vi "ADC SNR_Sweep_original.vi"(8 "error in (no error)":errorcluster, 9 "Sequence parameters":string[][](array[string])=[["Min limit", "Max limit", "Register sheet file", "Register Sheet"], ["", "", "CC2600.xls", "TX_BLE;Trim"], ["Reg write (addr;value)", "Operating frequency [Hz]", "", ""], ["NA", "2.44G", "", ""]], 10 "Run type":i32, 11 "Method parameters":T2={"Dev"={"Do not disturb DUT"=FALSE, "XOSC"=32000000.0, "Board type"="", "EM"="", "Configure tempboard"=TRUE, "Device specific info"=[], "Generic Object"=refnum}, "Method"={"Run type"=1, "Test name"="Current LPM2 4", "Comment"="", "Results folder"="", "AFC"=enum."Off", "Method name"="Current LPM2 4", "Method results"={"Excel brief report"=FALSE, "Spotfire report"=FALSE, "Starfish report"=FALSE}, "Operator"="", "Reference time"=timestamp(0 s since 1904-01-01), "AFC delay"=0.0, "Initialization"=enum."Enabled", "MD5 Sum"="", "HW addon board"=enum."None", "AFC Regsheet"="", "AFC Regfile"=path "", "dummy"=0.0}, "Inst"={"Instr"={"PS1"={"Name"="", "GPIB address"="", "VISA session"=""}, "PS2"={"Name"="", "GPIB address"="", "VISA session"=""}, "TC1"={"Name"="", "GPIB address"="", "VISA session"=""}, "TC2"={"Name"="", "GPIB address"="", "VISA session"=""}, "SA1"={"Name"="", "GPIB address"="", "VISA session"=""}, "SA2"={"Name"="", "GPIB address"="", "VISA session"=""}, "SG1"={"Name"="", "GPIB address"="", "VISA session"=""}, "SG2"={"Name"="", "GPIB address"="", "VISA session"=""}, "SG3"={"Name"="", "GPIB address"="", "VISA session"=""}, "MI1"={"Name"="", "GPIB address"="", "VISA session"=""}, "MI2"={"Name"="", "GPIB address"="", "VISA session"=""}, "SW SA"={"Name"="", "Controller addr"=""}, "SW SG"={"Name"="", "Controller addr"=""}, "MI3"={"Name"="", "GPIB address"="", "VISA session"=""}}, "Switchbox"={"RF Path"=0, "Cal compensation"=enum."TX", "Switchbox gain mode"="", "State"=enum."TX"}, "Instr to control (i.e. SA1)"="Default", "Intrument info string"=""}, "Sequence parameters"=[["Weight", "Min Limit", "Max Limit", "Register Sheet", "", "", "", "", "", "", "", "", ""], ["Vital", "", "1", "LPM2", "", "", "", "", "", "", "", "", ""], ["Resolution", "Reg write (addr;value)", "Chip mode", "Range", "", "", "", "", "", "", "", "", ""], ["u", "NA", "", "auto", "", "", "", "", "", "", "", "", ""]], "Cond"={"Temp logged"=25.0, "VDD1_PS1_6V"=-999.0, "VDD2_PS1_25V"=-999.0, "VDD4_PS2_25V"=-999.0, "VDD3_PS2_6V"=-999.0}, "Meas config"={"X-axis inner loop index"=32000000, "Y-axis outer loop index"=32000000, "X-axis"=[], "Y-axis"=[], "X-axis array req size"=32000000, "Y-axis array req size"=32000000, "Param description"=[], "Use meas clust for reporting"=FALSE, "Parameter index (page)"=0, "X-axis name"="", "Y-axis name"=""}} {"Cond"."VDD3_PS2_6V" format="%.3f"; "Cond"."VDD4_PS2_25V" format="%.3f"; "Cond"."VDD2_PS1_25V" format="%.3f"; "Cond"."VDD1_PS1_6V" format="%.3f"; "Method"."dummy" format="%.1p"; "Method"."AFC delay" format="%.1p"; "Dev"."XOSC" format="%.3p"}) -> (0 "Error Out":errorcluster[](array[cluster]), 1 "End Method Error":T2[](array[typedef]) {"Cond"."VDD3_PS2_6V" format="%.3f"; "Cond"."VDD4_PS2_25V" format="%.3f"; "Cond"."VDD2_PS1_25V" format="%.3f"; "Cond"."VDD1_PS1_6V" format="%.3f"; "Method"."dummy" format="%.1p"; "Method"."AFC delay" format="%.1p"; "Dev"."XOSC" format="%.3p"}, 2 "Short Results":string[](array[string]), 3 "Result summary":string[][](array[string])=[["Critical", "Output Power@2405 MHz", "-3", "4", "dBm"], ["Critical", "Output Power@2410 MHz", "-3", "4", "dBm"]])   [LabVIEW 2019]
doc: "[AutoDocStart]Performs crystal accuracy measurements. Measures the offset from ideal frequency. Primarily used for tuning XOSC capacitors and verifying XOSC trims.\n\nSweeping parameters: operating frequency, OSC override value and VDDR level\n\nResults: Offset frequency in ppm[AutoDocEnd]"
uses:
  User Lib/Generic chip methods/Classes/Generic_EM/Chameleon/Loki/Loki.lvclass
  User Lib/Generic chip methods/Classes/Generic_EM/Generic_EM/Generic_EM.lvclass
  1131283d-b54a-4ae3-ad67-71ff8f51acfe.vi
  3aacce8f-890b-4d9f-8ed2-28f84894822b.vi
  b456e919-2776-4fbb-a2ba-e4feed106c64.vi
  User Lib/Utilities/Cluster definitions/DUT VDD4.ctl
  User Lib/Utilities/Cluster definitions/DUT VDD3.ctl
  User Lib/Utilities/Cluster definitions/DUT VDD2.ctl
  User Lib/Utilities/Cluster definitions/DUT VDD1.ctl
  User Lib/Utilities/Cluster definitions/DUT vdd control.ctl
  69b5c8be-48d6-4f50-bcce-2a9f07fdba1a.vi
  User Lib/Utilities/Cluster definitions/Instr clust.ctl
  User Lib/Utilities/Cluster definitions/Method input.ctl
  User Lib/Utilities/Controls/Automatic Frequency Compensation types.ctl
  User Lib/Utilities/Controls/Method Reports.ctl
  User Lib/Utilities/Cluster definitions/Device specific info.ctl
  User Lib/Utilities/Cluster definitions/Method Initialization.ctl
  User Lib/Utilities/Switchbox control/SwitchBox_State._ENUMctl.ctl
  User Lib/Utilities/Controls/HW addon boards.ctl
panel:
  out "Output Response [All DUTs] 7":u32[][](array[numeric])
  out "Dynamic Parameters 4":T1={"SNR"=nan, "SNRD"=nan, "THD"=nan, "ENOB (SNRD)"=nan, "SFDR"=nan, "ENOB (SNR)"=nan, "Noise Power"=nan, "Signal power"=nan} {"Signal power" format="%.6f"; "Noise Power" format="%.2f"; "ENOB (SNR)" format="%.2f"; "SFDR" format="%.2f"; "ENOB (SNRD)" format="%.2f"; "THD" format="%.2f"; "SNRD" format="%.2f"; "SNR" format="%.2f"}
  out "detected Throughput":dbl=200065.4236150998
  out "Output Response [All DUTs] 6":u32[][](array[numeric])
  out "Dynamic Parameters 3":T1={"SNR"=nan, "SNRD"=nan, "THD"=nan, "ENOB (SNRD)"=nan, "SFDR"=nan, "ENOB (SNR)"=nan, "Noise Power"=nan, "Signal power"=nan} {"Signal power" format="%.6f"; "Noise Power" format="%.2f"; "ENOB (SNR)" format="%.2f"; "SFDR" format="%.2f"; "ENOB (SNRD)" format="%.2f"; "THD" format="%.2f"; "SNRD" format="%.2f"; "SNR" format="%.2f"}
  out "detected Throughput":dbl=200065.4236150998
  out "Output Response [All DUTs] 5":u32[][](array[numeric])
  out "Dynamic Parameters 2":T1={"SNR"=nan, "SNRD"=nan, "THD"=nan, "ENOB (SNRD)"=nan, "SFDR"=nan, "ENOB (SNR)"=nan, "Noise Power"=nan, "Signal power"=nan} {"Signal power" format="%.6f"; "Noise Power" format="%.2f"; "ENOB (SNR)" format="%.2f"; "SFDR" format="%.2f"; "ENOB (SNRD)" format="%.2f"; "THD" format="%.2f"; "SNRD" format="%.2f"; "SNR" format="%.2f"}
  out "detected Throughput":dbl=200065.4236150998
  out "detected Throughput":dbl=200065.4236150998
  out "Dynamic Parameters":T1={"SNR"=nan, "SNRD"=nan, "THD"=nan, "ENOB (SNRD)"=nan, "SFDR"=nan, "ENOB (SNR)"=nan, "Noise Power"=nan, "Signal power"=nan} {"Signal power" format="%.6f"; "Noise Power" format="%.2f"; "ENOB (SNR)" format="%.2f"; "SFDR" format="%.2f"; "ENOB (SNRD)" format="%.2f"; "THD" format="%.2f"; "SNRD" format="%.2f"; "SNR" format="%.2f"}
  out "Output Response [All DUTs] 4":u32[][](array[numeric])
  in  "Tab Control":T10(tab)
  # "°C"
  # "°C"
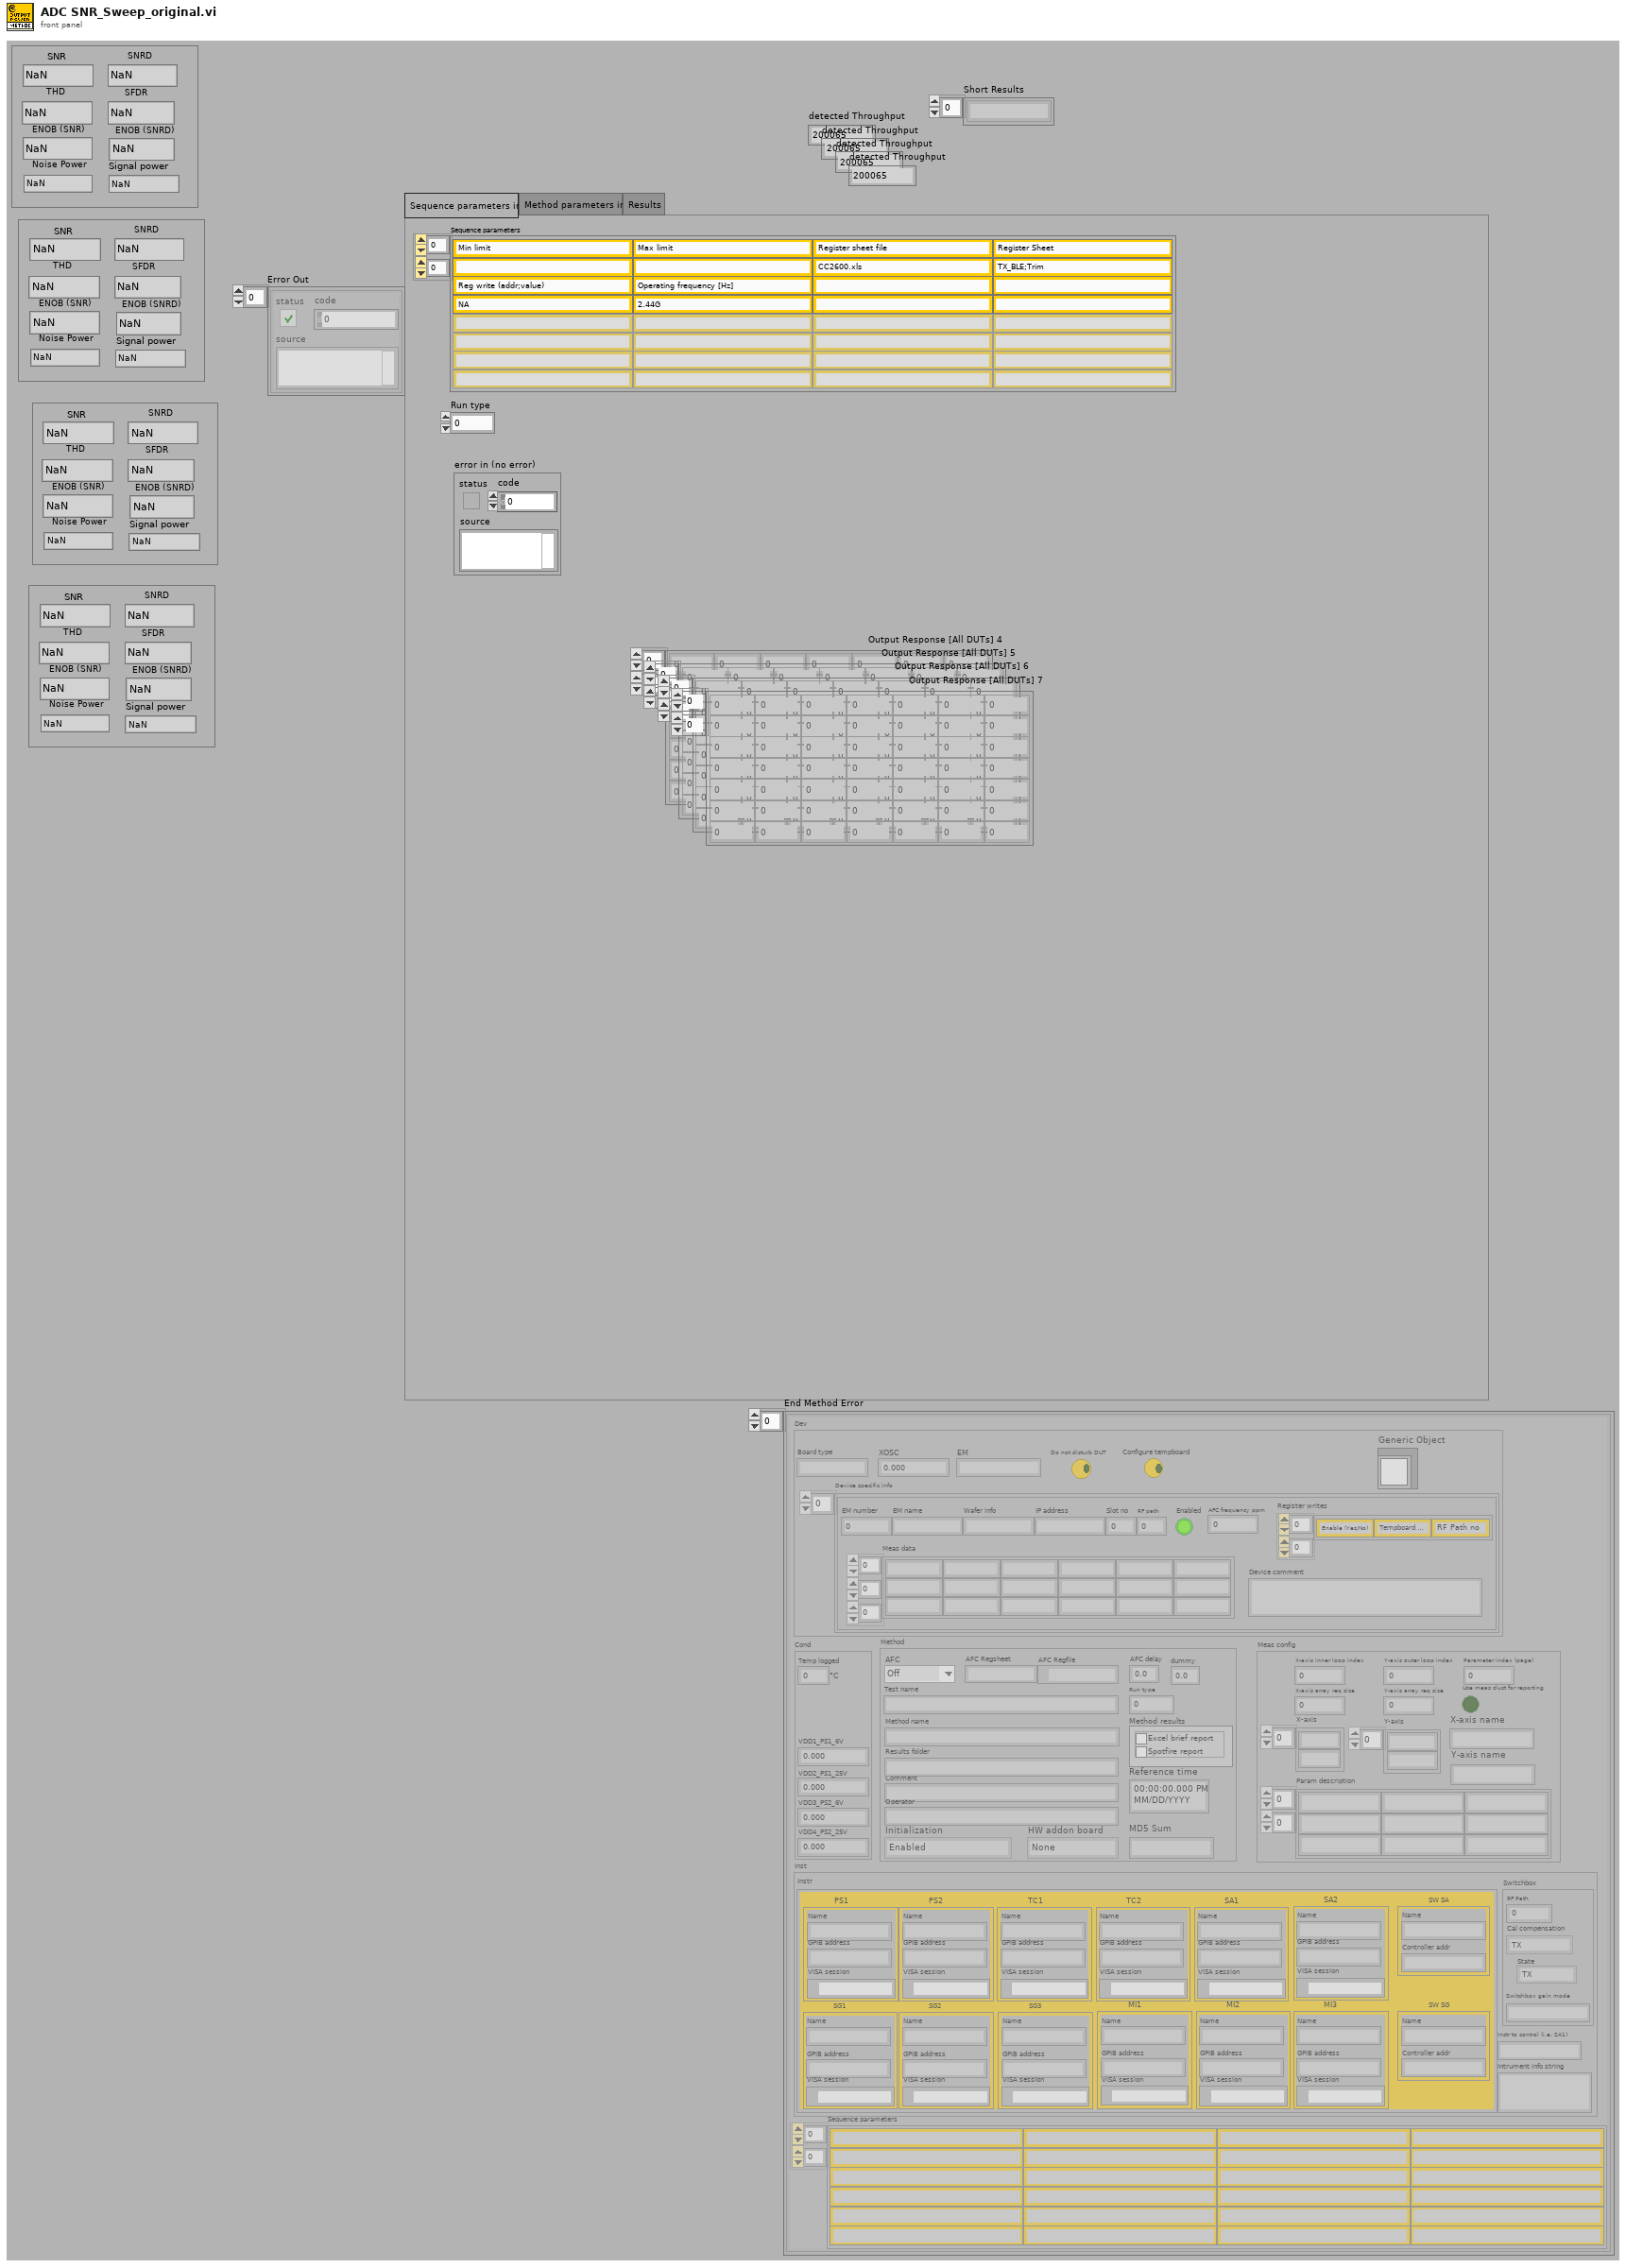
[diagram p1: front panel]
types:
  T1 = cluster{"SNR":dbl, "SNRD":dbl, "THD":dbl, "ENOB (SNRD)":dbl, "SFDR":dbl, "ENOB (SNR)":dbl, "Noise Power":dbl, "Signal power":dbl}
  T2 = typedef "Method input.ctl" = cluster{"Dev":cluster{"Do not disturb DUT":bool, "XOSC":dbl, "Board type":string, "EM":string, "Configure tempboard":bool, "Device specific info":T3[], "Generic Object":refnum<class>}, "Method":cluster{"Run type":i32, "Test name":string, "Comment":string, "Results folder":string, "AFC":T4, "Method name":string, "Method results":T5, "Operator":string, "Reference time":timestamp, "AFC delay":dbl, "Initialization":T6, "MD5 Sum":string, "HW addon board":T7, "AFC Regsheet":string, "AFC Regfile":path, "dummy":dbl}, "Inst":T8, "Sequence parameters":string[][], "Cond":cluster{"Temp logged":dbl, "VDD1_PS1_6V":dbl, "VDD2_PS1_25V":dbl, "VDD4_PS2_25V":dbl, "VDD3_PS2_6V":dbl}, "Meas config":cluster{"X-axis inner loop index":i32, "Y-axis outer loop index":i32, "X-axis":string[], "Y-axis":string[], "X-axis array req size":i32, "Y-axis array req size":i32, "Param description":string[][], "Use meas clust for reporting":bool, "Parameter index (page)":i32, "X-axis name":string, "Y-axis name":string}}
  T3 = typedef "Device specific info.ctl" = cluster{"EM number":u8, "IP address":string, "Enabled":bool, "Slot no":u8, "RF path":u8, "EM name":string, "Wafer info":string, "AFC frequency ppm":dbl, "Register writes":string[][], "Meas data":string[][][], "Device comment":string}
  T4 = typedef "Automatic Frequency Compensation types.ctl" = enum16{"Off", "Compensate Instrument frequency", "Compensate DUT frequency", "Predictive - Compensate Instrument frequency", "Predictive - Compensate DUT frequency", "Do not skip re-init - Compensate Instrument frequency", "Do not skip re-init - Compensate DUT frequency"}
  T5 = typedef "Method Reports.ctl" = cluster{"Excel brief report":bool, "Spotfire report":bool, "Starfish report":bool}
  T6 = typedef "Method Initialization.ctl" = enum16{"Enabled", "Skip Instr and Device Init", "Enabled with Separate Flash", "Set PS, Device Init and Skip Instr Init", "Skip Device Init"}
  T7 = typedef "HW addon boards.ctl" = enum16{"None", "Current meas 5EM", "Stresstest 10EM"}
  T8 = typedef "Instr clust.ctl" = cluster{"Instr":cluster{"PS1":cluster{"Name":string, "GPIB address":string, "VISA session":refnum<visa-resource-name>}, "PS2":cluster{"Name":string, "GPIB address":string, "VISA session":refnum<visa-resource-name>}, "TC1":cluster{"Name":string, "GPIB address":string, "VISA session":refnum<visa-resource-name>}, "TC2":cluster{"Name":string, "GPIB address":string, "VISA session":refnum<visa-resource-name>}, "SA1":cluster{"Name":string, "GPIB address":string, "VISA session":refnum<visa-resource-name>}, "SA2":cluster{"Name":string, "GPIB address":string, "VISA session":refnum<visa-resource-name>}, "SG1":cluster{"Name":string, "GPIB address":string, "VISA session":refnum<visa-resource-name>}, "SG2":cluster{"Name":string, "GPIB address":string, "VISA session":refnum<visa-resource-name>}, "SG3":cluster{"Name":string, "GPIB address":string, "VISA session":refnum<visa-resource-name>}, "MI1":cluster{"Name":string, "GPIB address":string, "VISA session":refnum<visa-resource-name>}, "MI2":cluster{"Name":string, "GPIB address":string, "VISA session":refnum<visa-resource-name>}, "SW SA":cluster{"Name":string, "Controller addr":string}, "SW SG":cluster{"Name":string, "Controller addr":string}, "MI3":cluster{"Name":string, "GPIB address":string, "VISA session":refnum<visa-resource-name>}}, "Switchbox":cluster{"RF Path":i32, "Cal compensation":enum16{"TX", "RX", "Interferer", "No compensation", "Interferer2"}, "Switchbox gain mode":string, "State":T9}, "Instr to control (i.e. SA1)":string, "Intrument info string":string}
  T9 = typedef "SwitchBox_State._ENUMctl.ctl" = enum16{"TX", "RX", "SP:TX", "SP:RX", "SW:TX", "SW:RX"}
  T10 = enum32{"Sequence parameters in", "Method parameters in", "Results"}
  T11 = typedef "DUT vdd control.ctl" = cluster{"VDD4 config":T12, "VDD3 config":T13, "VDD2 config":T14, "VDD1 config":T15}
  T12 = typedef "DUT VDD4.ctl" = u16
  T13 = typedef "DUT VDD3.ctl" = u16
  T14 = typedef "DUT VDD2.ctl" = u16
  T15 = typedef "DUT VDD1.ctl" = u16
  T16 = cluster{"Fundamental Frequency":dbl, "Sampling Frequncy":dbl, "No of Harmonics":u8, "Window":enum16{"None ", "Hanning", "Hamming", "Blackman-Harris", "Exact Blackman", "Blackman", "Flat Top", "4 Term B-Harris ", "7 Term B-Harris"}, "Blackman (fundamental power) bins)":dbl}
  T17 = enum32{"NI Card Settings", "Memory Read Setting", "DC Capture", "ADC Ramp", "ADC Sine", "SNR", "Cap Calibration"}
  T18 = enum32{"Read from Memory", "Read .dat file", "NI Card Capture", "None"}
  T19 = typedef "TFW ResponseData.ctl" = cluster{"errorCode":u32, "executionTime":u32, "processedCmdWord":u32, "responsePar":u32[], "actionCode":u32, "cmdStatus":u16}
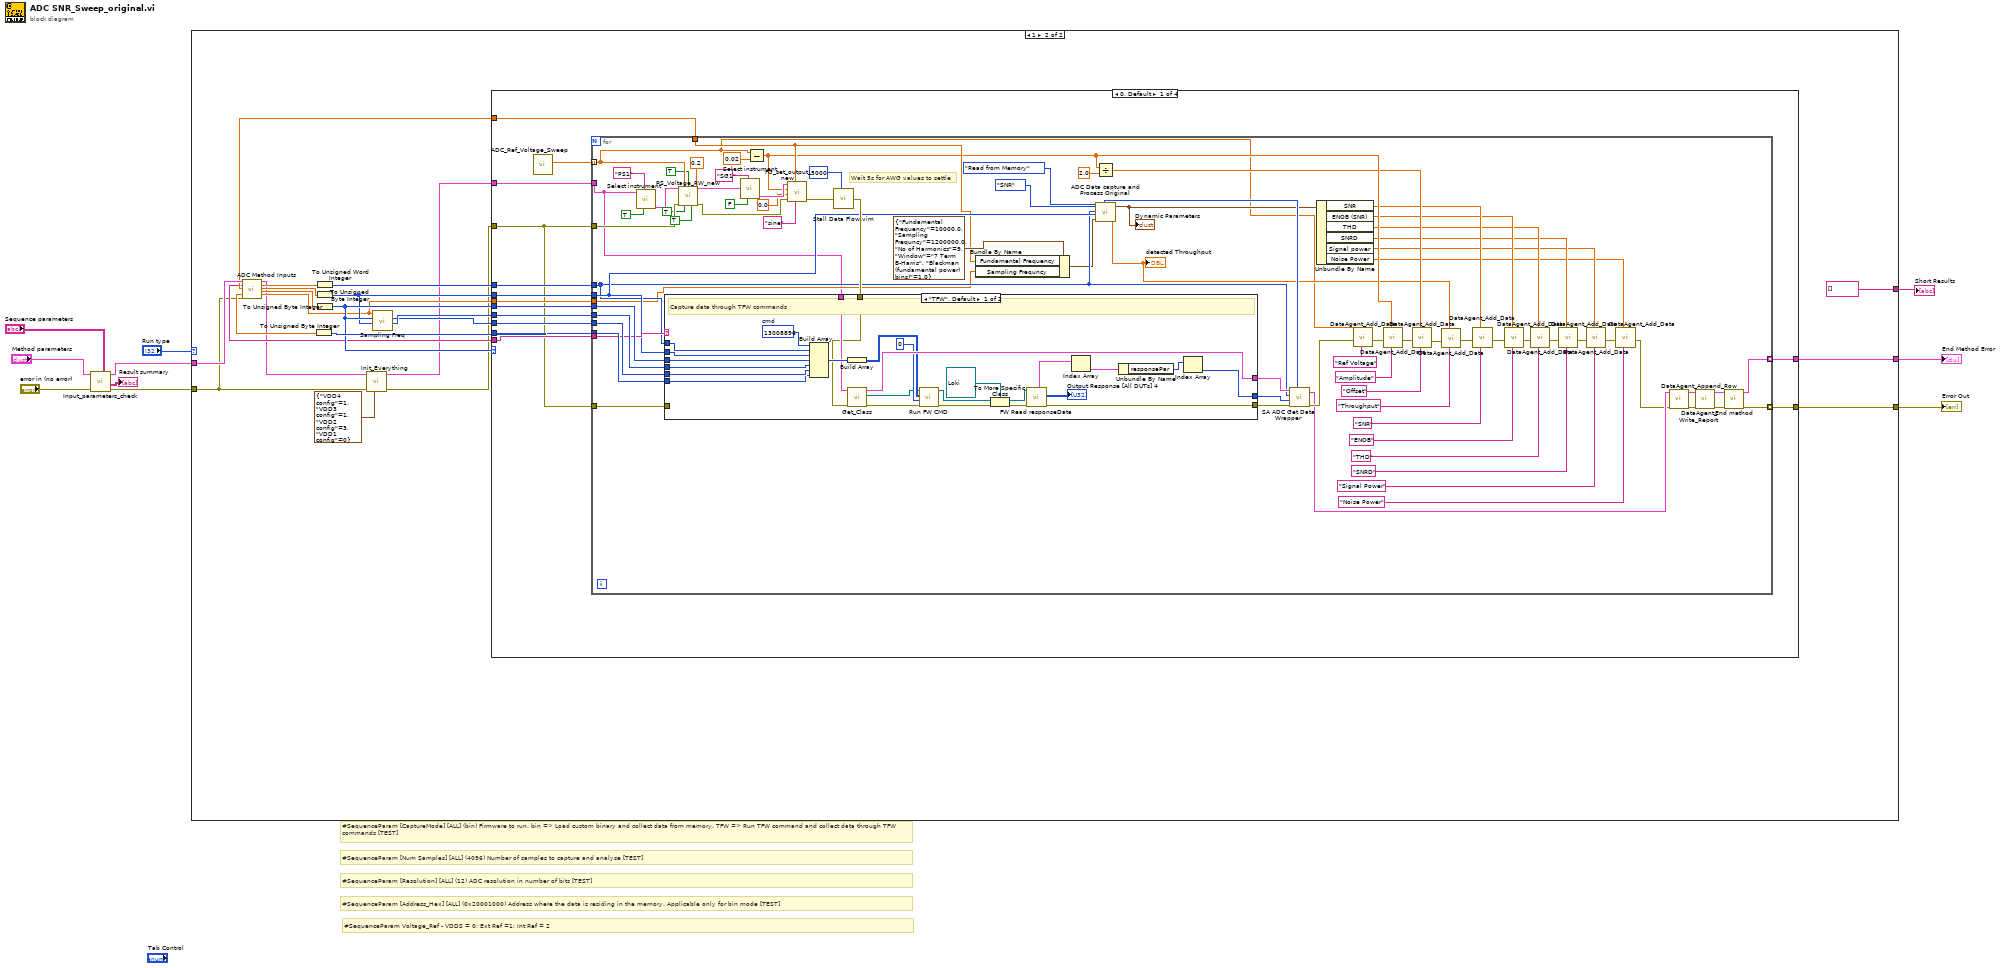
[diagram p0: block diagram]
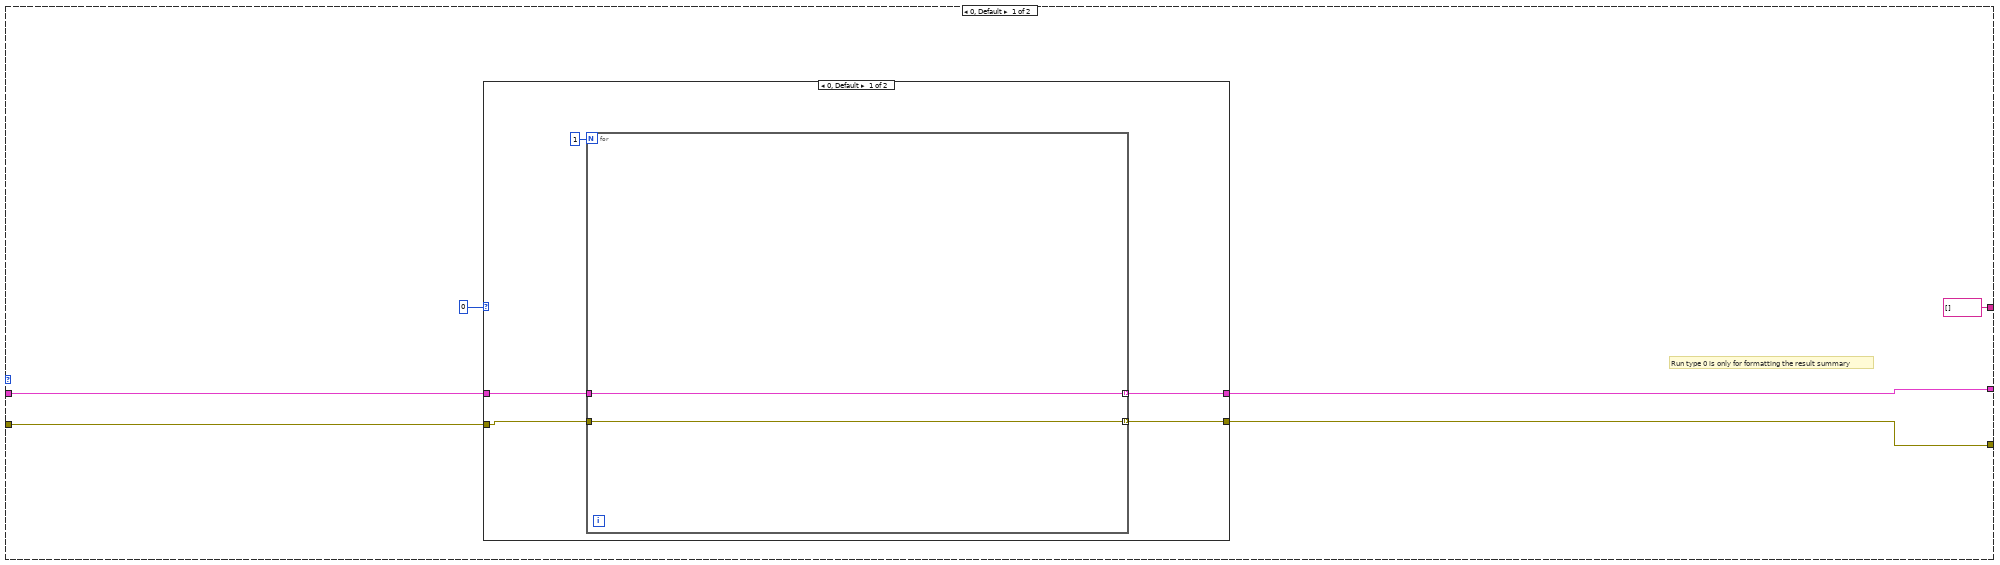
[diagram p2: hidden frame]
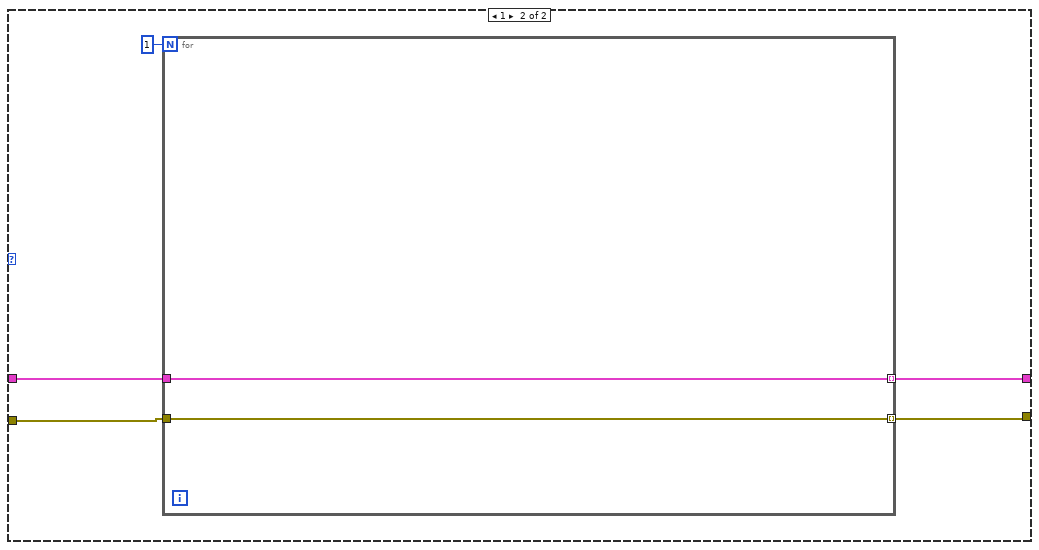
[diagram p3: hidden frame]
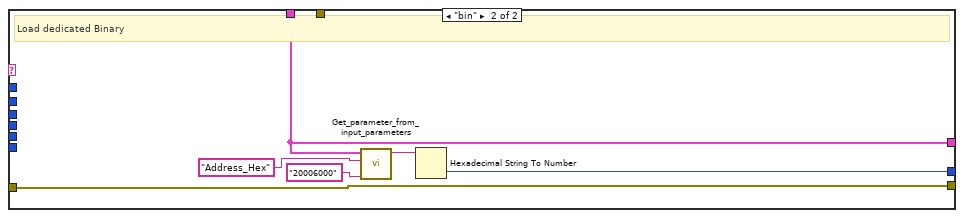
[diagram p4: hidden frame]
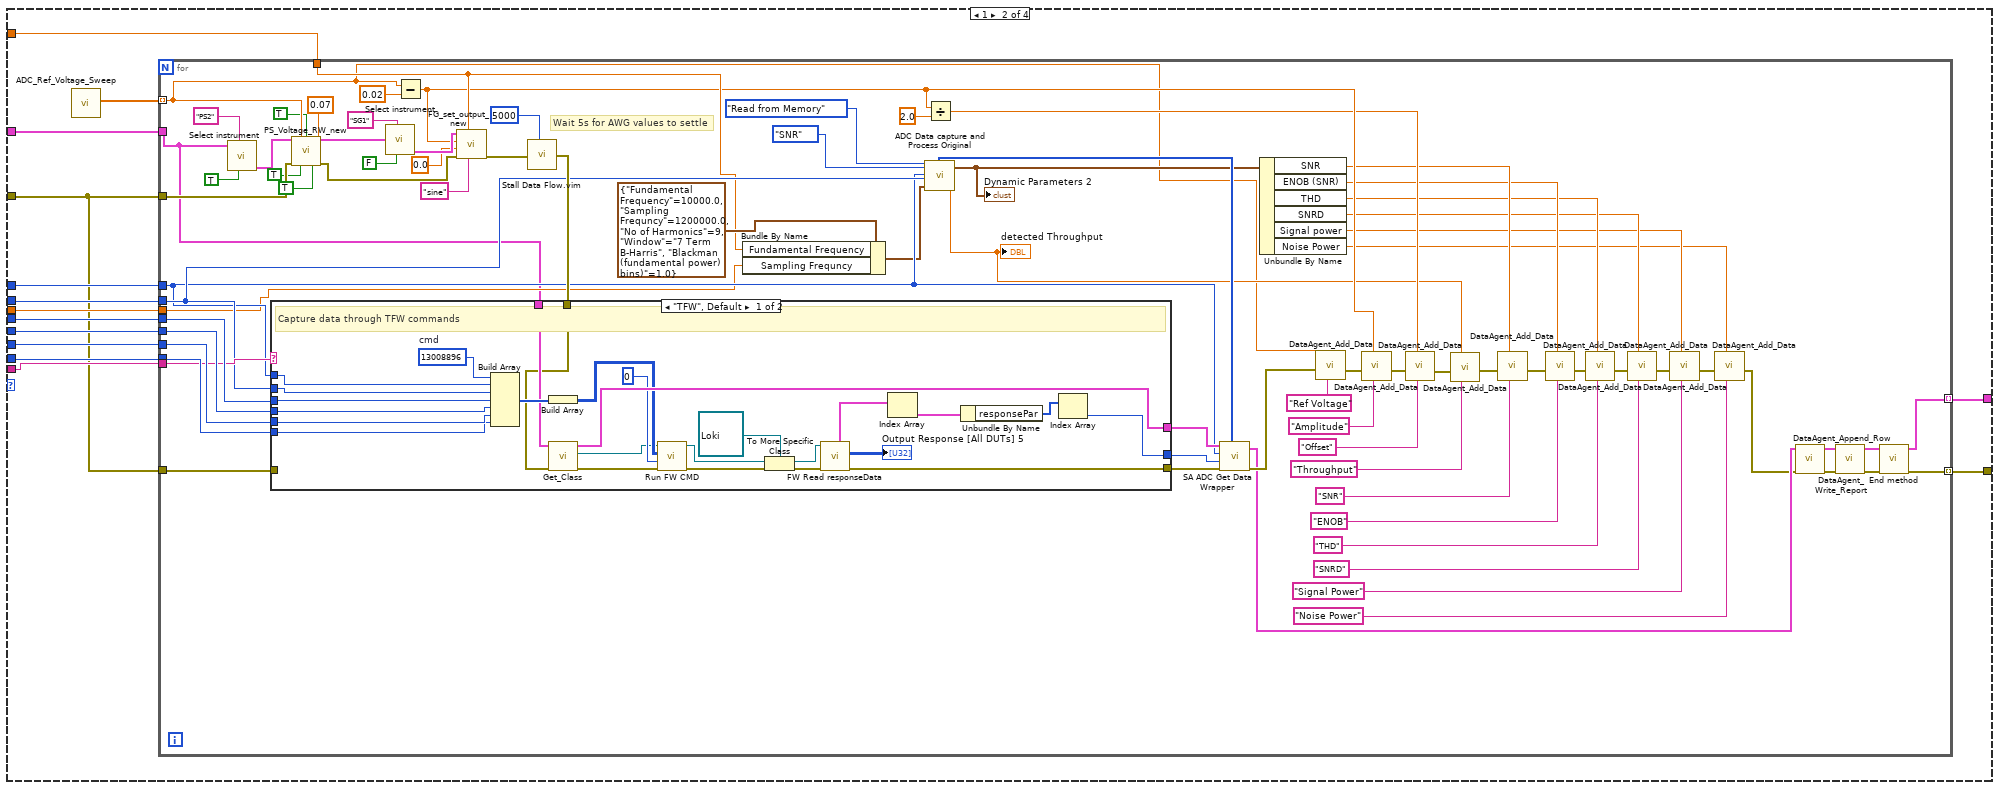
[diagram p5: hidden frame]
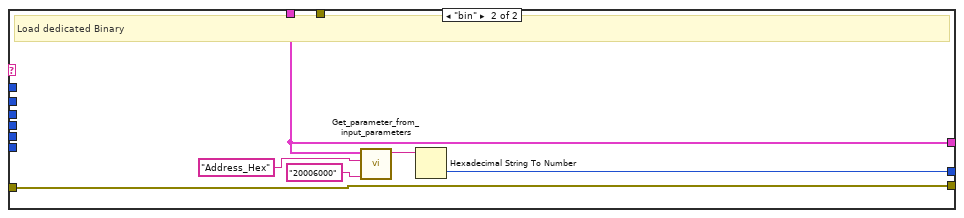
[diagram p6: hidden frame]
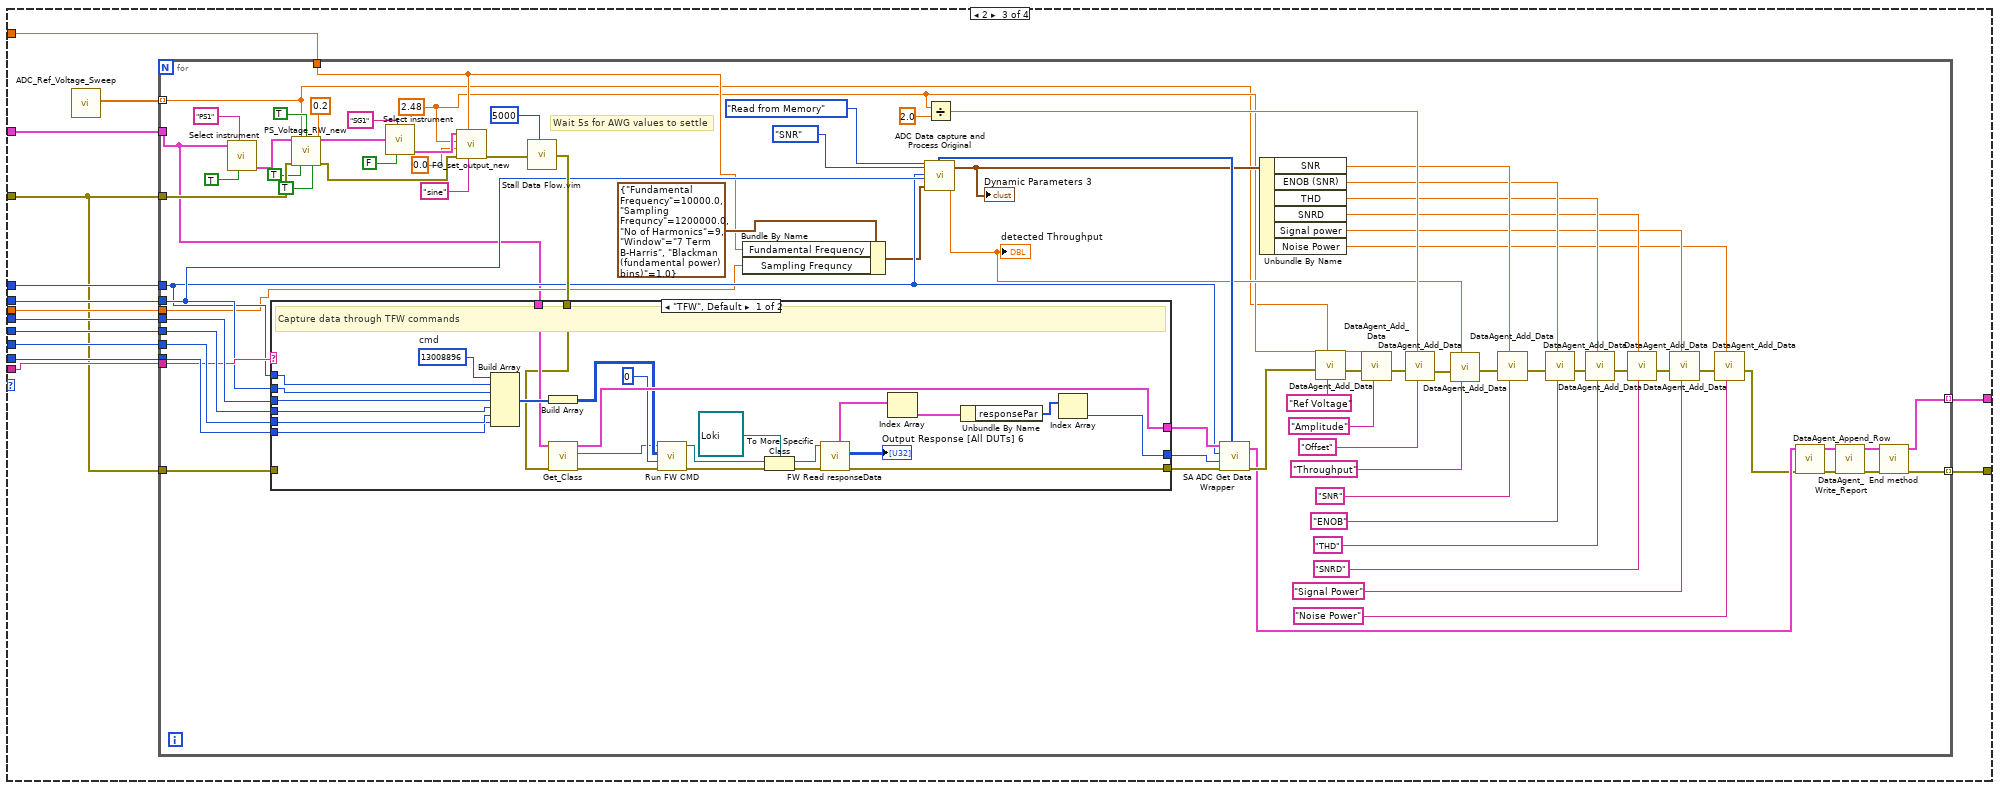
[diagram p7: hidden frame]
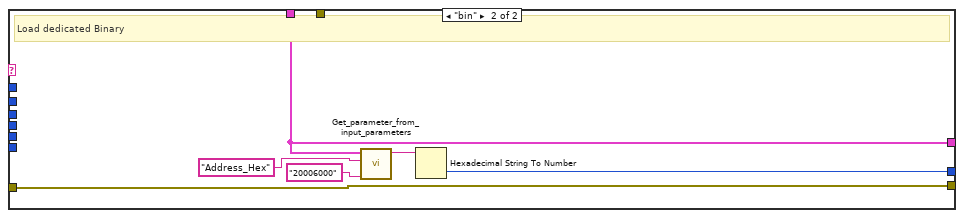
[diagram p8: hidden frame]
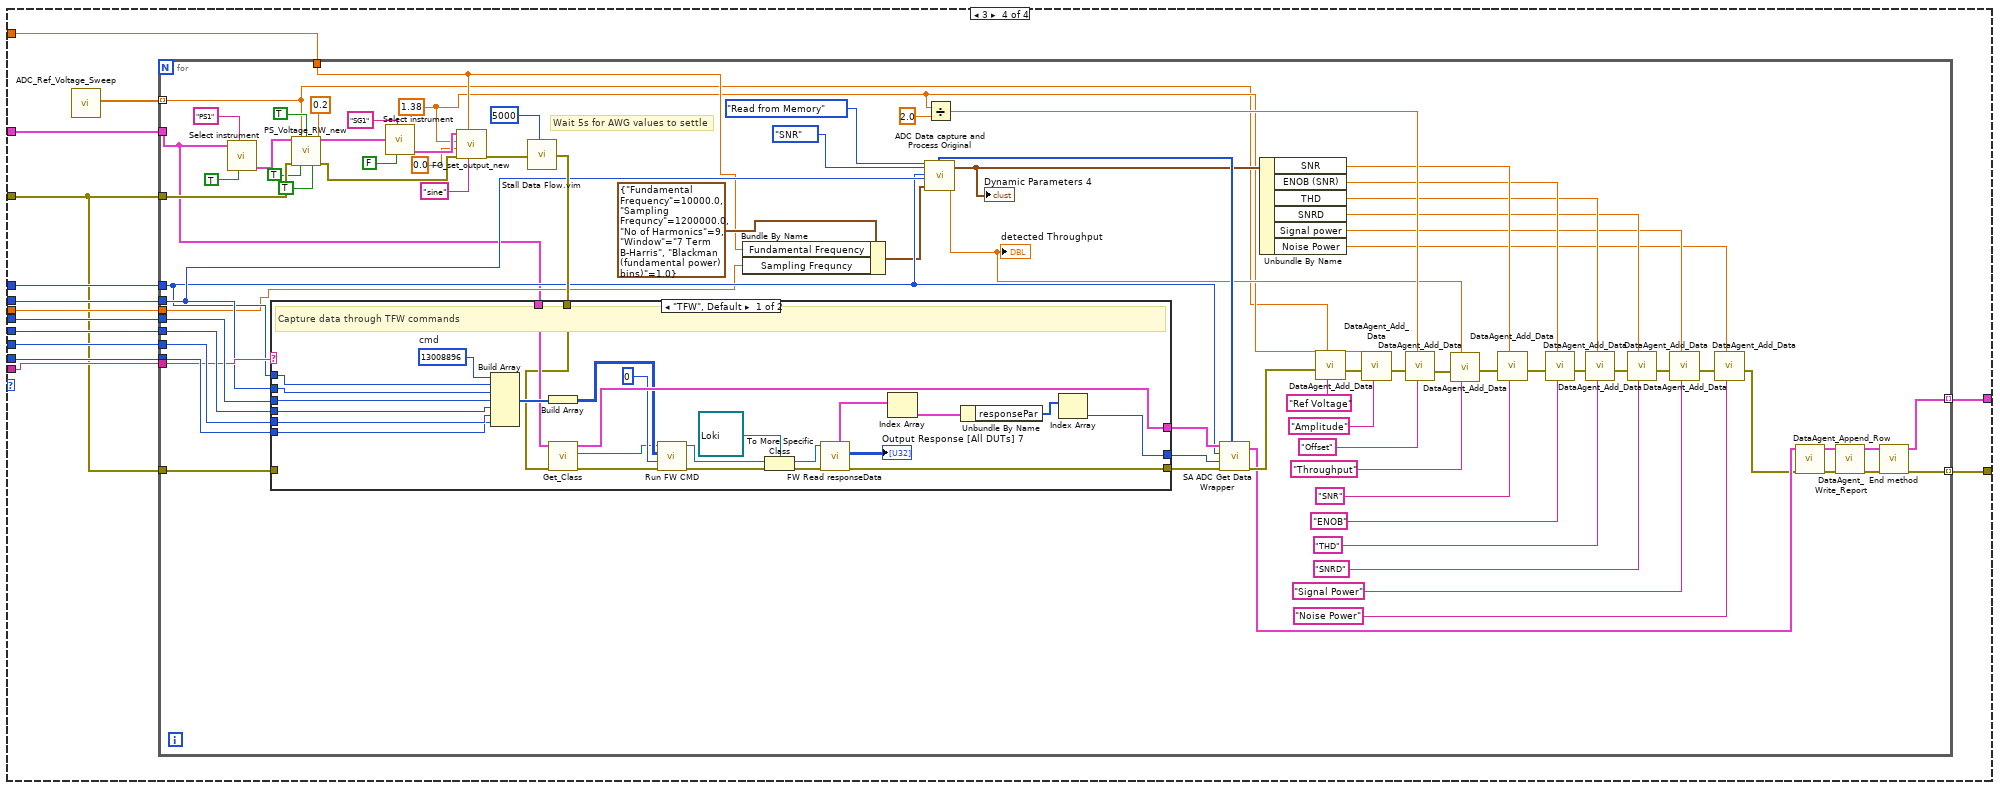
[diagram p9: hidden frame]
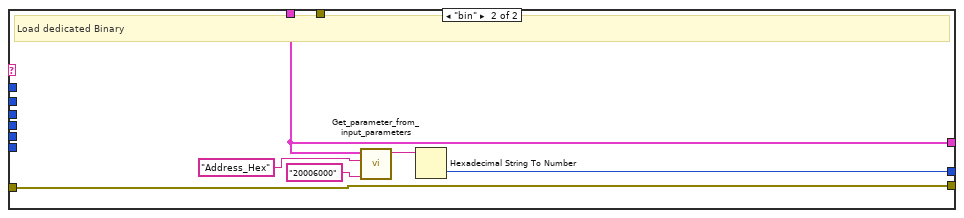
[diagram p10: hidden frame]
diagram:
  # "#SequenceParam Voltage_Ref - VDDS = 0; Ext Ref =1; Int Ref = 2"
  # "#SequenceParam [Num Samples] [ALL] (4096) Number of samples to capture and analyse [TEST]"
  # "#SequenceParam [CaptureMode] [ALL] (bin) Firmware to run. bin => Load custom binary and collect data from memory. TFW => Run TFW command and collect data through TFW commands [TEST]"
  # "#SequenceParam [Address_Hex] [ALL] (0x20001000) Address where the data is residing in the memory. Applicable only for bin mode [TEST]"
  # "#SequenceParam [Resolution] [ALL] (12) ADC resolution in number of bits [TEST]"
  n1 = call "Input_parameters_check.vi"("Sequence parameters"="Sequence parameters", "error in"="error in (no error)", "Method cluster in"="Method parameters") -> ("error out"=w10:errorcluster, "Result summary"=→"Result summary":string[][], "Method cluster out"=w6:T2)  [unwired: 6 in]
  n2 = case shown="1" "Run type" {
    tunnel: w10 -> [w12 w36]
    tunnel: w6 -> [w13 w52]
    tunnel: [w16 w38] -> w3
    tunnel: [w15 w37] -> w2
    tunnel: [string[] [] string[] []] -> w1
    frame 0, Default {
      # "Run type 0 is only for formatting the result summary"
      n3 = case shown="0, Default" 0 {
        tunnel: w13 -> [w21 w28]
        tunnel: w12 -> [w18 w27]
        tunnel: [w20 w26] -> w16
        tunnel: [w19 w25] -> w15
        frame 0, Default {
          n4 = for {
            N: 1 -> [_]
            tunnel: w21 -> [w23]
            tunnel: [w23] -> w20 mode=indexing
            tunnel: [w22] -> w19 mode=indexing
            tunnel: w18 -> [w22]
          }
        }
        frame 1 {
          n5 = for {
            N: 1 -> [_]
            tunnel: w28 -> [w30]
            tunnel: w27 -> [w29]
            tunnel: [w30] -> w26 mode=indexing
            tunnel: [w29] -> w25 mode=indexing
          }
        }
      }
    }
    frame 1 {
      n6 = call "ADC Method Inputs.vi"("Method cluster in"=w52, "error in (no error)"=w36) -> ("Capture Mode"=w40:string, "Signal Freq"=w43:dbl, "ADC Channel No."=w48:dbl, "Method cluster out"=w35:T2, "Num Samples"=w51:dbl, "Resolution"=w50:dbl, "Voltage Ref"=w49:dbl, "Sampling Freq"=w39:dbl)  [unwired: 6 in, 4 out]
      n7 = To Unsigned Byte Integer(number=w48) -> (unsigned 8bit integer=w44:u8)
      n8 = To Unsigned Byte Integer(number=w50) -> (unsigned 8bit integer=w41:u8)
      n9 = To Unsigned Byte Integer(number=w49) -> (unsigned 8bit integer=w42:u8)
      n10 = To Unsigned Word Integer(number=w51) -> (unsigned 16bit integer=w47:u16)
      n11 = call "Init_Everything.vi"("VDD config"=T11 {"VDD4 config"=1, "VDD3 config"=1, "VDD2 config"=3, "VDD1 config"=0}, "error in"=w36, "Method cluster In"=w35) -> ("error out"=w33:errorcluster, "Method cluster out"=w34:T2)  [unwired: 5 in, 2 out]
      n12 = call "Sampling Freq.vi"("Resolution"=w41, "Voltage Ref"=w42, "Sampling Freq"=w39) -> ("LGPT Count"=w46:u16, "SCOMP"=w45:u16)  [unwired: 7 in]
      n13 = case shown="0, Default" w42 {
        tunnel: w47 -> [w66 w190 w314 w437]
        tunnel: w41 -> [w65 w189 w313 w436]
        tunnel: w42 -> [w64 w188 w312 w435]
        tunnel: w46 -> [w63 w187 w311 w434]
        tunnel: w45 -> [w62 w186 w310 w433]
        tunnel: w44 -> [w61 w185 w309 w432]
        tunnel: w34 -> [w59 w183 w307 w430]
        tunnel: w33 -> [w53 w177 w301 w424]
        tunnel: w43 -> [w58 w182 w306 w429]
        tunnel: w40 -> [w57 w181 w305 w428]
        tunnel: w39 -> [w56 w180 w304 w427]
        tunnel: [w55 w179 w303 w426] -> w37
        tunnel: [w54 w178 w302 w425] -> w38
        frame 0, Default {
          n14 = call "ADC_Ref_Voltage_Sweep.vi"() -> ("Ref voltage sweep"=w60:dbl[])  [unwired: 11 in]
          n15 = for {
            tunnel: w66 -> [w121]
            tunnel: w65 -> [w122]
            tunnel: w64 -> [w141]
            tunnel: w63 -> [w140]
            tunnel: w62 -> [w139]
            tunnel: w61 -> [w138]
            tunnel: w57 -> [w137]
            tunnel: w60 -> [w70] mode=indexing
            tunnel: w59 -> [w68]
            tunnel: w53 -> [w76]
            tunnel: w58 -> [w118]
            tunnel: w56 -> [w117]
            tunnel: [w79] -> w55 mode=indexing
            tunnel: [w78] -> w54 mode=indexing
            tunnel: w53 -> [w77]
            # "Wait 5s for AWG values to settle"
            n16 = call "Select instrument.vi"("Method cluster (T) / Instr cluster (F)"=TRUE, "Instr.Instr to control (i.e. SA1)"="PS1", "Method cluster in"=w68) -> ("Instr out"=w73:T8)  [unwired: 6 in, 2 out]
            n17 = call "PS_Voltage_RW_new.vi"("InstrCluster in"=w73, "Set Voltage"=w70, "Limit to 4V (T)"=TRUE, "Current(0)"=0.2, "error in (no error)"=w76, "Off (F)                         On (T)"=TRUE, "Read (F)                      Write (T)"=TRUE) -> ("InstrCluster out"=w74:T8, "error out"=w75:errorcluster)  [unwired: 6 in, 1 out]
            n18 = call "Select instrument.vi"("Method cluster (T) / Instr cluster (F)"=FALSE, "Instr.Instr to control (i.e. SA1)"="SG1", "Instr in"=w74) -> ("Instr out"=w131:T8)  [unwired: 6 in, 2 out]
            n19 = Subtract(x=w70, y=0.02) -> (x-y=w98:dbl)
            n20 = call "FG_set_output_new.vi"("Function (DC, Sine, Square, Triangle, Ramp up, Ramp down, Pulse)"="sine", "Frequency [Hz]"=w118, "error in"=w75, "Low voltage"=0.0, "High voltage (or DC)"=w98, "InstrCluster in"=w131) -> ("error out"=w128:errorcluster)  [unwired: 4 in, 1 out]
            n21 = call "Stall Data Flow.vim"("value in"=w128, "milliseconds to wait"=u32 5000) -> ("value out"=w127:errorcluster)  [unwired: 1 out]
            n22 = case shown="\"TFW\", Default" w137 {
              tunnel: [w170 w171] -> w144
              tunnel: [w165 w172] -> w143
              tunnel: [w153 w173] -> w142
              tunnel: w121 -> [w152 _]
              tunnel: w122 -> [w151 _]
              tunnel: w141 -> [w150 _]
              tunnel: w140 -> [w149 _]
              tunnel: w139 -> [w148 _]
              tunnel: w138 -> [w147 _]
              tunnel: w68 -> [w146 w171]
              tunnel: w127 -> [w145 _]
              tunnel: w77 -> [_ w172]
              frame "TFW", Default {
                w168 = u32 13008896  # cmd
                # "Capture data through TFW commands"
                n23 = Build Array(w168, w152, w151, w150, w149, w148, w147) -> (w167:u32[])
                n24 = Build Array(w167) -> (w166:u32[][])
                n25 = call "Get_Class.vi"("error in (no error)"=w145, "Method cluster in"=w146) -> ("error out"=w163:errorcluster, "Class Out"=w162:refnum<class "Generic_EM.lvclass">, "Method cluster out"=w170:T2)  [unwired: 6 in, 1 out]
                n26 = call-dynamic "Run FW CMD.vi"("error in (no error)"=w163, "Handler"=u8 0, "cmdBuf"=w166, "Generic_EM in"=w162) -> ("error out"=w158:errorcluster, "Generic_EM out"=w161:refnum<class "Generic_EM.lvclass">)  [unwired: 6 in]
                n27 = To More Specific Class(target class=refnum<class "Loki.lvclass"> refnum ("Loki in"), reference=w161, error in=w158) -> (specific class reference=w159:refnum<class "Loki.lvclass">, error out=w157:errorcluster)
                n28 = call "FW Read responseData.vi"("error in (no error)"=w157, "Loki in"=w159) -> ("error out"=w165:errorcluster, "Output Response [All DUTs]"=→"Output Response [All DUTs] 4":u32[][], "Response"=w155:T19[])  [unwired: 6 in, 1 out]
                n29 = Index Array(array=w155) -> (element=w156:T19)  [unwired: 1 in]
                n30 = Unbundle By Name(w156) -> ("responsePar"=w154:u32[])
                n31 = Index Array(array=w154) -> (element=w153:u32)  [unwired: 1 in]
              }
              frame "bin" {
                # "Load dedicated Binary"
                n32 = call "Get_parameter_from_input_parameters.vi"("Default value (used if not specified on Front Panel)"="20006000", "Parameter name"="Address_Hex" ("SA_ param name"), "Method cluster (if input param empty)"=w171) -> ("value as String"=w176:string)  [unwired: 2 in, 6 out]
                n33 = Hexadecimal String To Number(string=w176) -> (number=w173:u32)  [unwired: 2 in, 1 out]
              }
            }
            n34 = Bundle By Name(cluster=T16 {"Fundamental Frequency"=10000.0, "Sampling Frequncy"=1200000.0, "No of Harmonics"=9, "Window"=enum."7 Term B-Harris", "Blackman (fundamental power) bins)"=1.0} ("Inputs for Dyanmic para"), "Fundamental Frequency"=w118, "Sampling Frequncy"=w117) -> (w119:T16)
            n35 = Divide(x=w98, y=2.0) -> (x/y=w96:dbl)
            n36 = call "SA ADC Get Data Wrapper.vi"("error in"=w143, "Data Address"=w142, "Num Samples"=w121, "Method cluster in"=w144) -> ("error out"=w88:errorcluster, "output cluster"=w81:T2, "Output in mV"=w123:u32[])  [unwired: 2 in, 3 out]
            n37 = call "ADC Data capture and Process Original.vi"("ADC Output Read Method"=T18."Read from Memory", "Select the Tab to project"=T17."SNR", "No.of samples(SNR)"=w121, "Resolution"=w122, "Inputs for Dyanmic para"=w119, "Waveform"=w123) -> ("detected Throughput"=w95:dbl, "Dynamic Parameters"=w116:T1)  [unwired: 15 in, 5 out]
            "Dynamic Parameters" <- w116
            "detected Throughput" <- w95
            n38 = Unbundle By Name(w116) -> ("SNR"=w94:dbl, "ENOB (SNR)"=w93:dbl, "THD"=w92:dbl, "SNRD"=w91:dbl, "Signal power"=w90:dbl, "Noise Power"=w89:dbl)
            n39 = call "DataAgent_Add_Data.vi"("ColumnName"="Ref Voltage", "Data"=w70, "error in (no error)"=w88) -> ("error out"=w86:errorcluster)  [unwired: 8 in]
            n40 = call "DataAgent_Add_Data.vi"("ColumnName"="Amplitude" ("Default Value"), "Data"=w98, "error in (no error)"=w86) -> ("error out"=w114:errorcluster)  [unwired: 8 in]
            n41 = call "DataAgent_Add_Data.vi"("ColumnName"="Offset" ("Default Value"), "Data"=w96, "error in (no error)"=w114) -> ("error out"=w100:errorcluster)  [unwired: 8 in]
            n42 = call "DataAgent_Add_Data.vi"("ColumnName"="Throughput", "Data"=w95, "error in (no error)"=w100) -> ("error out"=w99:errorcluster)  [unwired: 8 in]
            n43 = call "DataAgent_Add_Data.vi"("ColumnName"="SNR", "Data"=w94, "error in (no error)"=w99) -> ("error out"=w112:errorcluster)  [unwired: 8 in]
            n44 = call "DataAgent_Add_Data.vi"("ColumnName"="ENOB", "Data"=w93, "error in (no error)"=w112) -> ("error out"=w107:errorcluster)  [unwired: 8 in]
            n45 = call "DataAgent_Add_Data.vi"("ColumnName"="THD", "Data"=w92, "error in (no error)"=w107) -> ("error out"=w106:errorcluster)  [unwired: 8 in]
            n46 = call "DataAgent_Add_Data.vi"("ColumnName"="SNRD", "Data"=w91, "error in (no error)"=w106) -> ("error out"=w105:errorcluster)  [unwired: 8 in]
            n47 = call "DataAgent_Add_Data.vi"("ColumnName"="Signal Power", "Data"=w90, "error in (no error)"=w105) -> ("error out"=w102:errorcluster)  [unwired: 8 in]
            n48 = call "DataAgent_Add_Data.vi"("ColumnName"="Noise Power", "Data"=w89, "error in (no error)"=w102) -> ("error out"=w80:errorcluster)  [unwired: 8 in]
            n49 = call "DataAgent_Append_Row.vi"("error in (no error)"=w80, "Method cluster in"=w81) -> ("error out"=w82:errorcluster, "Method cluster out"=w83:T2)  [unwired: 8 in]
            n50 = call "DataAgent_Write_Report.vi"("error in (no error)"=w82, "Method cluster in"=w83) -> ("error out"=w85:errorcluster, "Method cluster out"=w84:T2)  [unwired: 8 in]
            n51 = call "End method.vi"("error in"=w85, "Method cluster in"=w84) -> ("error out"=w79:errorcluster, "Method cluster out"=w78:T2)  [unwired: 7 in, 1 out]
          }
        }
        frame 1 {
          n52 = call "ADC_Ref_Voltage_Sweep.vi"() -> ("Ref voltage sweep"=w184:dbl[])  [unwired: 11 in]
          n53 = for {
            tunnel: w190 -> [w245]
            tunnel: w189 -> [w246]
            tunnel: w188 -> [w265]
            tunnel: w187 -> [w264]
            tunnel: w186 -> [w263]
            tunnel: w185 -> [w262]
            tunnel: w181 -> [w261]
            tunnel: w184 -> [w194] mode=indexing
            tunnel: w183 -> [w192]
            tunnel: w177 -> [w200]
            tunnel: w182 -> [w242]
            tunnel: w180 -> [w241]
            tunnel: [w203] -> w179 mode=indexing
            tunnel: [w202] -> w178 mode=indexing
            tunnel: w177 -> [w201]
            # "Wait 5s for AWG values to settle"
            n54 = call "Select instrument.vi"("Method cluster (T) / Instr cluster (F)"=TRUE, "Instr.Instr to control (i.e. SA1)"="PS2", "Method cluster in"=w192) -> ("Instr out"=w197:T8)  [unwired: 6 in, 2 out]
            n55 = call "PS_Voltage_RW_new.vi"("InstrCluster in"=w197, "Set Voltage"=w194, "Limit to 4V (T)"=TRUE, "Current(0)"=0.07, "error in (no error)"=w200, "Off (F)                         On (T)"=TRUE, "Read (F)                      Write (T)"=TRUE) -> ("InstrCluster out"=w198:T8, "error out"=w199:errorcluster)  [unwired: 6 in, 1 out]
            n56 = call "Select instrument.vi"("Method cluster (T) / Instr cluster (F)"=FALSE, "Instr.Instr to control (i.e. SA1)"="SG1", "Instr in"=w198) -> ("Instr out"=w255:T8)  [unwired: 6 in, 2 out]
            n57 = Subtract(x=w194, y=0.02) -> (x-y=w222:dbl)
            n58 = call "FG_set_output_new.vi"("Function (DC, Sine, Square, Triangle, Ramp up, Ramp down, Pulse)"="sine", "Frequency [Hz]"=w242, "error in"=w199, "Low voltage"=0.0, "High voltage (or DC)"=w222, "InstrCluster in"=w255) -> ("error out"=w252:errorcluster)  [unwired: 4 in, 1 out]
            n59 = call "Stall Data Flow.vim"("value in"=w252, "milliseconds to wait"=u32 5000) -> ("value out"=w251:errorcluster)  [unwired: 1 out]
            n60 = case shown="\"TFW\", Default" w261 {
              tunnel: [w294 w295] -> w268
              tunnel: [w289 w296] -> w267
              tunnel: [w277 w297] -> w266
              tunnel: w245 -> [w276 _]
              tunnel: w246 -> [w275 _]
              tunnel: w265 -> [w274 _]
              tunnel: w264 -> [w273 _]
              tunnel: w263 -> [w272 _]
              tunnel: w262 -> [w271 _]
              tunnel: w192 -> [w270 w295]
              tunnel: w251 -> [w269 _]
              tunnel: w201 -> [_ w296]
              frame "TFW", Default {
                w292 = u32 13008896  # cmd
                # "Capture data through TFW commands"
                n61 = Build Array(w292, w276, w275, w274, w273, w272, w271) -> (w291:u32[])
                n62 = Build Array(w291) -> (w290:u32[][])
                n63 = call "Get_Class.vi"("error in (no error)"=w269, "Method cluster in"=w270) -> ("error out"=w287:errorcluster, "Class Out"=w286:refnum<class "Generic_EM.lvclass">, "Method cluster out"=w294:T2)  [unwired: 6 in, 1 out]
                n64 = call-dynamic "Run FW CMD.vi"("error in (no error)"=w287, "Handler"=u8 0, "cmdBuf"=w290, "Generic_EM in"=w286) -> ("error out"=w282:errorcluster, "Generic_EM out"=w285:refnum<class "Generic_EM.lvclass">)  [unwired: 6 in]
                n65 = To More Specific Class(target class=refnum<class "Loki.lvclass"> refnum ("Loki in"), reference=w285, error in=w282) -> (specific class reference=w283:refnum<class "Loki.lvclass">, error out=w281:errorcluster)
                n66 = call "FW Read responseData.vi"("error in (no error)"=w281, "Loki in"=w283) -> ("error out"=w289:errorcluster, "Output Response [All DUTs]"=→"Output Response [All DUTs] 5":u32[][], "Response"=w279:T19[])  [unwired: 6 in, 1 out]
                n67 = Index Array(array=w279) -> (element=w280:T19)  [unwired: 1 in]
                n68 = Unbundle By Name(w280) -> ("responsePar"=w278:u32[])
                n69 = Index Array(array=w278) -> (element=w277:u32)  [unwired: 1 in]
              }
              frame "bin" {
                # "Load dedicated Binary"
                n70 = call "Get_parameter_from_input_parameters.vi"("Default value (used if not specified on Front Panel)"="20006000", "Parameter name"="Address_Hex" ("SA_ param name"), "Method cluster (if input param empty)"=w295) -> ("value as String"=w300:string)  [unwired: 2 in, 6 out]
                n71 = Hexadecimal String To Number(string=w300) -> (number=w297:u32)  [unwired: 2 in, 1 out]
              }
            }
            n72 = Bundle By Name(cluster=T16 {"Fundamental Frequency"=10000.0, "Sampling Frequncy"=1200000.0, "No of Harmonics"=9, "Window"=enum."7 Term B-Harris", "Blackman (fundamental power) bins)"=1.0} ("Inputs for Dyanmic para"), "Fundamental Frequency"=w242, "Sampling Frequncy"=w241) -> (w243:T16)
            n73 = Divide(x=w222, y=2.0) -> (x/y=w220:dbl)
            n74 = call "SA ADC Get Data Wrapper.vi"("error in"=w267, "Data Address"=w266, "Num Samples"=w245, "Method cluster in"=w268) -> ("error out"=w212:errorcluster, "output cluster"=w205:T2, "Output in mV"=w247:u32[])  [unwired: 2 in, 3 out]
            n75 = call "ADC Data capture and Process Original.vi"("ADC Output Read Method"=T18."Read from Memory", "Select the Tab to project"=T17."SNR", "No.of samples(SNR)"=w245, "Resolution"=w246, "Inputs for Dyanmic para"=w243, "Waveform"=w247) -> ("detected Throughput"=w219:dbl, "Dynamic Parameters"=w240:T1)  [unwired: 15 in, 5 out]
            "Dynamic Parameters 2" <- w240
            "detected Throughput" <- w219
            n76 = Unbundle By Name(w240) -> ("SNR"=w218:dbl, "ENOB (SNR)"=w217:dbl, "THD"=w216:dbl, "SNRD"=w215:dbl, "Signal power"=w214:dbl, "Noise Power"=w213:dbl)
            n77 = call "DataAgent_Add_Data.vi"("ColumnName"="Ref Voltage", "Data"=w194, "error in (no error)"=w212) -> ("error out"=w210:errorcluster)  [unwired: 8 in]
            n78 = call "DataAgent_Add_Data.vi"("ColumnName"="Amplitude" ("Default Value"), "Data"=w222, "error in (no error)"=w210) -> ("error out"=w238:errorcluster)  [unwired: 8 in]
            n79 = call "DataAgent_Add_Data.vi"("ColumnName"="Offset" ("Default Value"), "Data"=w220, "error in (no error)"=w238) -> ("error out"=w224:errorcluster)  [unwired: 8 in]
            n80 = call "DataAgent_Add_Data.vi"("ColumnName"="Throughput", "Data"=w219, "error in (no error)"=w224) -> ("error out"=w223:errorcluster)  [unwired: 8 in]
            n81 = call "DataAgent_Add_Data.vi"("ColumnName"="SNR", "Data"=w218, "error in (no error)"=w223) -> ("error out"=w236:errorcluster)  [unwired: 8 in]
            n82 = call "DataAgent_Add_Data.vi"("ColumnName"="ENOB", "Data"=w217, "error in (no error)"=w236) -> ("error out"=w231:errorcluster)  [unwired: 8 in]
            n83 = call "DataAgent_Add_Data.vi"("ColumnName"="THD", "Data"=w216, "error in (no error)"=w231) -> ("error out"=w230:errorcluster)  [unwired: 8 in]
            n84 = call "DataAgent_Add_Data.vi"("ColumnName"="SNRD", "Data"=w215, "error in (no error)"=w230) -> ("error out"=w229:errorcluster)  [unwired: 8 in]
            n85 = call "DataAgent_Add_Data.vi"("ColumnName"="Signal Power", "Data"=w214, "error in (no error)"=w229) -> ("error out"=w226:errorcluster)  [unwired: 8 in]
            n86 = call "DataAgent_Add_Data.vi"("ColumnName"="Noise Power", "Data"=w213, "error in (no error)"=w226) -> ("error out"=w204:errorcluster)  [unwired: 8 in]
            n87 = call "DataAgent_Append_Row.vi"("error in (no error)"=w204, "Method cluster in"=w205) -> ("error out"=w206:errorcluster, "Method cluster out"=w207:T2)  [unwired: 8 in]
            n88 = call "DataAgent_Write_Report.vi"("error in (no error)"=w206, "Method cluster in"=w207) -> ("error out"=w209:errorcluster, "Method cluster out"=w208:T2)  [unwired: 8 in]
            n89 = call "End method.vi"("error in"=w209, "Method cluster in"=w208) -> ("error out"=w203:errorcluster, "Method cluster out"=w202:T2)  [unwired: 7 in, 1 out]
          }
        }
        frame 2 {
          n90 = call "ADC_Ref_Voltage_Sweep.vi"() -> ("Ref voltage sweep"=w308:dbl[])  [unwired: 11 in]
          n91 = for {
            tunnel: w314 -> [w369]
            tunnel: w313 -> [w370]
            tunnel: w312 -> [w388]
            tunnel: w311 -> [w387]
            tunnel: w310 -> [w386]
            tunnel: w309 -> [w385]
            tunnel: w305 -> [w384]
            tunnel: w308 -> [w316] mode=indexing
            tunnel: w307 -> [w318]
            tunnel: w301 -> [w325]
            tunnel: w306 -> [w366]
            tunnel: w304 -> [w365]
            tunnel: [w328] -> w303 mode=indexing
            tunnel: [w327] -> w302 mode=indexing
            tunnel: w301 -> [w326]
            w317 = 2.48 ("High voltage (or DC)")
            # "Wait 5s for AWG values to settle"
            n92 = call "Select instrument.vi"("Method cluster (T) / Instr cluster (F)"=TRUE, "Instr.Instr to control (i.e. SA1)"="PS1", "Method cluster in"=w318) -> ("Instr out"=w322:T8)  [unwired: 6 in, 2 out]
            n93 = call "PS_Voltage_RW_new.vi"("InstrCluster in"=w322, "Set Voltage"=w316, "Limit to 4V (T)"=TRUE, "Current(0)"=0.2, "error in (no error)"=w325, "Off (F)                         On (T)"=TRUE, "Read (F)                      Write (T)"=TRUE) -> ("InstrCluster out"=w323:T8, "error out"=w324:errorcluster)  [unwired: 6 in, 1 out]
            n94 = call "Select instrument.vi"("Method cluster (T) / Instr cluster (F)"=FALSE, "Instr.Instr to control (i.e. SA1)"="SG1", "Instr in"=w323) -> ("Instr out"=w379:T8)  [unwired: 6 in, 2 out]
            n95 = call "FG_set_output_new.vi"("Function (DC, Sine, Square, Triangle, Ramp up, Ramp down, Pulse)"="sine", "Frequency [Hz]"=w366, "error in"=w324, "Low voltage"=0.0, "High voltage (or DC)"=w317, "InstrCluster in"=w379) -> ("error out"=w376:errorcluster)  [unwired: 4 in, 1 out]
            n96 = call "Stall Data Flow.vim"("value in"=w376, "milliseconds to wait"=u32 5000) -> ("value out"=w375:errorcluster)  [unwired: 1 out]
            n97 = case shown="\"TFW\", Default" w384 {
              tunnel: [w417 w418] -> w391
              tunnel: [w412 w419] -> w390
              tunnel: [w400 w420] -> w389
              tunnel: w369 -> [w399 _]
              tunnel: w370 -> [w398 _]
              tunnel: w388 -> [w397 _]
              tunnel: w387 -> [w396 _]
              tunnel: w386 -> [w395 _]
              tunnel: w385 -> [w394 _]
              tunnel: w318 -> [w393 w418]
              tunnel: w375 -> [w392 _]
              tunnel: w326 -> [_ w419]
              frame "TFW", Default {
                w415 = u32 13008896  # cmd
                # "Capture data through TFW commands"
                n98 = Build Array(w415, w399, w398, w397, w396, w395, w394) -> (w414:u32[])
                n99 = Build Array(w414) -> (w413:u32[][])
                n100 = call "Get_Class.vi"("error in (no error)"=w392, "Method cluster in"=w393) -> ("error out"=w410:errorcluster, "Class Out"=w409:refnum<class "Generic_EM.lvclass">, "Method cluster out"=w417:T2)  [unwired: 6 in, 1 out]
                n101 = call-dynamic "Run FW CMD.vi"("error in (no error)"=w410, "Handler"=u8 0, "cmdBuf"=w413, "Generic_EM in"=w409) -> ("error out"=w405:errorcluster, "Generic_EM out"=w408:refnum<class "Generic_EM.lvclass">)  [unwired: 6 in]
                n102 = To More Specific Class(target class=refnum<class "Loki.lvclass"> refnum ("Loki in"), reference=w408, error in=w405) -> (specific class reference=w406:refnum<class "Loki.lvclass">, error out=w404:errorcluster)
                n103 = call "FW Read responseData.vi"("error in (no error)"=w404, "Loki in"=w406) -> ("error out"=w412:errorcluster, "Output Response [All DUTs]"=→"Output Response [All DUTs] 6":u32[][], "Response"=w402:T19[])  [unwired: 6 in, 1 out]
                n104 = Index Array(array=w402) -> (element=w403:T19)  [unwired: 1 in]
                n105 = Unbundle By Name(w403) -> ("responsePar"=w401:u32[])
                n106 = Index Array(array=w401) -> (element=w400:u32)  [unwired: 1 in]
              }
              frame "bin" {
                # "Load dedicated Binary"
                n107 = call "Get_parameter_from_input_parameters.vi"("Default value (used if not specified on Front Panel)"="20006000", "Parameter name"="Address_Hex" ("SA_ param name"), "Method cluster (if input param empty)"=w418) -> ("value as String"=w423:string)  [unwired: 2 in, 6 out]
                n108 = Hexadecimal String To Number(string=w423) -> (number=w420:u32)  [unwired: 2 in, 1 out]
              }
            }
            n109 = Bundle By Name(cluster=T16 {"Fundamental Frequency"=10000.0, "Sampling Frequncy"=1200000.0, "No of Harmonics"=9, "Window"=enum."7 Term B-Harris", "Blackman (fundamental power) bins)"=1.0} ("Inputs for Dyanmic para"), "Fundamental Frequency"=w366, "Sampling Frequncy"=w365) -> (w367:T16)
            n110 = Divide(x=w317, y=2.0) -> (x/y=w345:dbl)
            n111 = call "SA ADC Get Data Wrapper.vi"("error in"=w390, "Data Address"=w389, "Num Samples"=w369, "Method cluster in"=w391) -> ("error out"=w337:errorcluster, "output cluster"=w330:T2, "Output in mV"=w371:u32[])  [unwired: 2 in, 3 out]
            n112 = call "ADC Data capture and Process Original.vi"("ADC Output Read Method"=T18."Read from Memory", "Select the Tab to project"=T17."SNR", "No.of samples(SNR)"=w369, "Resolution"=w370, "Inputs for Dyanmic para"=w367, "Waveform"=w371) -> ("detected Throughput"=w344:dbl, "Dynamic Parameters"=w364:T1)  [unwired: 15 in, 5 out]
            "Dynamic Parameters 3" <- w364
            "detected Throughput" <- w344
            n113 = Unbundle By Name(w364) -> ("SNR"=w343:dbl, "ENOB (SNR)"=w342:dbl, "THD"=w341:dbl, "SNRD"=w340:dbl, "Signal power"=w339:dbl, "Noise Power"=w338:dbl)
            n114 = call "DataAgent_Add_Data.vi"("ColumnName"="Ref Voltage", "Data"=w316, "error in (no error)"=w337) -> ("error out"=w335:errorcluster)  [unwired: 8 in]
            n115 = call "DataAgent_Add_Data.vi"("ColumnName"="Amplitude" ("Default Value"), "Data"=w317, "error in (no error)"=w335) -> ("error out"=w362:errorcluster)  [unwired: 8 in]
            n116 = call "DataAgent_Add_Data.vi"("ColumnName"="Offset" ("Default Value"), "Data"=w345, "error in (no error)"=w362) -> ("error out"=w348:errorcluster)  [unwired: 8 in]
            n117 = call "DataAgent_Add_Data.vi"("ColumnName"="Throughput", "Data"=w344, "error in (no error)"=w348) -> ("error out"=w347:errorcluster)  [unwired: 8 in]
            n118 = call "DataAgent_Add_Data.vi"("ColumnName"="SNR", "Data"=w343, "error in (no error)"=w347) -> ("error out"=w360:errorcluster)  [unwired: 8 in]
            n119 = call "DataAgent_Add_Data.vi"("ColumnName"="ENOB", "Data"=w342, "error in (no error)"=w360) -> ("error out"=w355:errorcluster)  [unwired: 8 in]
            n120 = call "DataAgent_Add_Data.vi"("ColumnName"="THD", "Data"=w341, "error in (no error)"=w355) -> ("error out"=w354:errorcluster)  [unwired: 8 in]
            n121 = call "DataAgent_Add_Data.vi"("ColumnName"="SNRD", "Data"=w340, "error in (no error)"=w354) -> ("error out"=w353:errorcluster)  [unwired: 8 in]
            n122 = call "DataAgent_Add_Data.vi"("ColumnName"="Signal Power", "Data"=w339, "error in (no error)"=w353) -> ("error out"=w350:errorcluster)  [unwired: 8 in]
            n123 = call "DataAgent_Add_Data.vi"("ColumnName"="Noise Power", "Data"=w338, "error in (no error)"=w350) -> ("error out"=w329:errorcluster)  [unwired: 8 in]
            n124 = call "DataAgent_Append_Row.vi"("error in (no error)"=w329, "Method cluster in"=w330) -> ("error out"=w331:errorcluster, "Method cluster out"=w332:T2)  [unwired: 8 in]
            n125 = call "DataAgent_Write_Report.vi"("error in (no error)"=w331, "Method cluster in"=w332) -> ("error out"=w334:errorcluster, "Method cluster out"=w333:T2)  [unwired: 8 in]
            n126 = call "End method.vi"("error in"=w334, "Method cluster in"=w333) -> ("error out"=w328:errorcluster, "Method cluster out"=w327:T2)  [unwired: 7 in, 1 out]
          }
        }
        frame 3 {
          n127 = call "ADC_Ref_Voltage_Sweep.vi"() -> ("Ref voltage sweep"=w431:dbl[])  [unwired: 11 in]
          n128 = for {
            tunnel: w437 -> [w492]
            tunnel: w436 -> [w493]
            tunnel: w435 -> [w511]
            tunnel: w434 -> [w510]
            tunnel: w433 -> [w509]
            tunnel: w432 -> [w508]
            tunnel: w428 -> [w507]
            tunnel: w431 -> [w439] mode=indexing
            tunnel: w430 -> [w441]
            tunnel: w424 -> [w448]
            tunnel: w429 -> [w489]
            tunnel: w427 -> [w488]
            tunnel: [w451] -> w426 mode=indexing
            tunnel: [w450] -> w425 mode=indexing
            tunnel: w424 -> [w449]
            w440 = 1.38 ("High voltage (or DC)")
            # "Wait 5s for AWG values to settle"
            n129 = call "Select instrument.vi"("Method cluster (T) / Instr cluster (F)"=TRUE, "Instr.Instr to control (i.e. SA1)"="PS1", "Method cluster in"=w441) -> ("Instr out"=w445:T8)  [unwired: 6 in, 2 out]
            n130 = call "PS_Voltage_RW_new.vi"("InstrCluster in"=w445, "Set Voltage"=w439, "Limit to 4V (T)"=TRUE, "Current(0)"=0.2, "error in (no error)"=w448, "Off (F)                         On (T)"=TRUE, "Read (F)                      Write (T)"=TRUE) -> ("InstrCluster out"=w446:T8, "error out"=w447:errorcluster)  [unwired: 6 in, 1 out]
            n131 = call "Select instrument.vi"("Method cluster (T) / Instr cluster (F)"=FALSE, "Instr.Instr to control (i.e. SA1)"="SG1", "Instr in"=w446) -> ("Instr out"=w502:T8)  [unwired: 6 in, 2 out]
            n132 = call "FG_set_output_new.vi"("Function (DC, Sine, Square, Triangle, Ramp up, Ramp down, Pulse)"="sine", "Frequency [Hz]"=w489, "error in"=w447, "Low voltage"=0.0, "High voltage (or DC)"=w440, "InstrCluster in"=w502) -> ("error out"=w499:errorcluster)  [unwired: 4 in, 1 out]
            n133 = call "Stall Data Flow.vim"("value in"=w499, "milliseconds to wait"=u32 5000) -> ("value out"=w498:errorcluster)  [unwired: 1 out]
            n134 = case shown="\"TFW\", Default" w507 {
              tunnel: [w540 w541] -> w514
              tunnel: [w535 w542] -> w513
              tunnel: [w523 w543] -> w512
              tunnel: w492 -> [w522 _]
              tunnel: w493 -> [w521 _]
              tunnel: w511 -> [w520 _]
              tunnel: w510 -> [w519 _]
              tunnel: w509 -> [w518 _]
              tunnel: w508 -> [w517 _]
              tunnel: w441 -> [w516 w541]
              tunnel: w498 -> [w515 _]
              tunnel: w449 -> [_ w542]
              frame "TFW", Default {
                w538 = u32 13008896  # cmd
                # "Capture data through TFW commands"
                n135 = Build Array(w538, w522, w521, w520, w519, w518, w517) -> (w537:u32[])
                n136 = Build Array(w537) -> (w536:u32[][])
                n137 = call "Get_Class.vi"("error in (no error)"=w515, "Method cluster in"=w516) -> ("error out"=w533:errorcluster, "Class Out"=w532:refnum<class "Generic_EM.lvclass">, "Method cluster out"=w540:T2)  [unwired: 6 in, 1 out]
                n138 = call-dynamic "Run FW CMD.vi"("error in (no error)"=w533, "Handler"=u8 0, "cmdBuf"=w536, "Generic_EM in"=w532) -> ("error out"=w528:errorcluster, "Generic_EM out"=w531:refnum<class "Generic_EM.lvclass">)  [unwired: 6 in]
                n139 = To More Specific Class(target class=refnum<class "Loki.lvclass"> refnum ("Loki in"), reference=w531, error in=w528) -> (specific class reference=w529:refnum<class "Loki.lvclass">, error out=w527:errorcluster)
                n140 = call "FW Read responseData.vi"("error in (no error)"=w527, "Loki in"=w529) -> ("error out"=w535:errorcluster, "Output Response [All DUTs]"=→"Output Response [All DUTs] 7":u32[][], "Response"=w525:T19[])  [unwired: 6 in, 1 out]
                n141 = Index Array(array=w525) -> (element=w526:T19)  [unwired: 1 in]
                n142 = Unbundle By Name(w526) -> ("responsePar"=w524:u32[])
                n143 = Index Array(array=w524) -> (element=w523:u32)  [unwired: 1 in]
              }
              frame "bin" {
                # "Load dedicated Binary"
                n144 = call "Get_parameter_from_input_parameters.vi"("Default value (used if not specified on Front Panel)"="20006000", "Parameter name"="Address_Hex" ("SA_ param name"), "Method cluster (if input param empty)"=w541) -> ("value as String"=w546:string)  [unwired: 2 in, 6 out]
                n145 = Hexadecimal String To Number(string=w546) -> (number=w543:u32)  [unwired: 2 in, 1 out]
              }
            }
            n146 = Bundle By Name(cluster=T16 {"Fundamental Frequency"=10000.0, "Sampling Frequncy"=1200000.0, "No of Harmonics"=9, "Window"=enum."7 Term B-Harris", "Blackman (fundamental power) bins)"=1.0} ("Inputs for Dyanmic para"), "Fundamental Frequency"=w489, "Sampling Frequncy"=w488) -> (w490:T16)
            n147 = Divide(x=w440, y=2.0) -> (x/y=w468:dbl)
            n148 = call "SA ADC Get Data Wrapper.vi"("error in"=w513, "Data Address"=w512, "Num Samples"=w492, "Method cluster in"=w514) -> ("error out"=w460:errorcluster, "output cluster"=w453:T2, "Output in mV"=w494:u32[])  [unwired: 2 in, 3 out]
            n149 = call "ADC Data capture and Process Original.vi"("ADC Output Read Method"=T18."Read from Memory", "Select the Tab to project"=T17."SNR", "No.of samples(SNR)"=w492, "Resolution"=w493, "Inputs for Dyanmic para"=w490, "Waveform"=w494) -> ("detected Throughput"=w467:dbl, "Dynamic Parameters"=w487:T1)  [unwired: 15 in, 5 out]
            "Dynamic Parameters 4" <- w487
            "detected Throughput" <- w467
            n150 = Unbundle By Name(w487) -> ("SNR"=w466:dbl, "ENOB (SNR)"=w465:dbl, "THD"=w464:dbl, "SNRD"=w463:dbl, "Signal power"=w462:dbl, "Noise Power"=w461:dbl)
            n151 = call "DataAgent_Add_Data.vi"("ColumnName"="Ref Voltage", "Data"=w439, "error in (no error)"=w460) -> ("error out"=w458:errorcluster)  [unwired: 8 in]
            n152 = call "DataAgent_Add_Data.vi"("ColumnName"="Amplitude" ("Default Value"), "Data"=w440, "error in (no error)"=w458) -> ("error out"=w485:errorcluster)  [unwired: 8 in]
            n153 = call "DataAgent_Add_Data.vi"("ColumnName"="Offset" ("Default Value"), "Data"=w468, "error in (no error)"=w485) -> ("error out"=w471:errorcluster)  [unwired: 8 in]
            n154 = call "DataAgent_Add_Data.vi"("ColumnName"="Throughput", "Data"=w467, "error in (no error)"=w471) -> ("error out"=w470:errorcluster)  [unwired: 8 in]
            n155 = call "DataAgent_Add_Data.vi"("ColumnName"="SNR", "Data"=w466, "error in (no error)"=w470) -> ("error out"=w483:errorcluster)  [unwired: 8 in]
            n156 = call "DataAgent_Add_Data.vi"("ColumnName"="ENOB", "Data"=w465, "error in (no error)"=w483) -> ("error out"=w478:errorcluster)  [unwired: 8 in]
            n157 = call "DataAgent_Add_Data.vi"("ColumnName"="THD", "Data"=w464, "error in (no error)"=w478) -> ("error out"=w477:errorcluster)  [unwired: 8 in]
            n158 = call "DataAgent_Add_Data.vi"("ColumnName"="SNRD", "Data"=w463, "error in (no error)"=w477) -> ("error out"=w476:errorcluster)  [unwired: 8 in]
            n159 = call "DataAgent_Add_Data.vi"("ColumnName"="Signal Power", "Data"=w462, "error in (no error)"=w476) -> ("error out"=w473:errorcluster)  [unwired: 8 in]
            n160 = call "DataAgent_Add_Data.vi"("ColumnName"="Noise Power", "Data"=w461, "error in (no error)"=w473) -> ("error out"=w452:errorcluster)  [unwired: 8 in]
            n161 = call "DataAgent_Append_Row.vi"("error in (no error)"=w452, "Method cluster in"=w453) -> ("error out"=w454:errorcluster, "Method cluster out"=w455:T2)  [unwired: 8 in]
            n162 = call "DataAgent_Write_Report.vi"("error in (no error)"=w454, "Method cluster in"=w455) -> ("error out"=w457:errorcluster, "Method cluster out"=w456:T2)  [unwired: 8 in]
            n163 = call "End method.vi"("error in"=w457, "Method cluster in"=w456) -> ("error out"=w451:errorcluster, "Method cluster out"=w450:T2)  [unwired: 7 in, 1 out]
          }
        }
      }
    }
  }
  "End Method Error" <- w3
  "Error Out" <- w2
  "Short Results" <- w1
